vi "SolutionCalculator (SubVI).vi"(3 "Iterative?":bool, 4 "Max Iteration Count":dbl=2.0, 5 "Base Run (matrix)":T1, 6 "Response Coefficients":cdb[][](array[numeric])) -> (0 "Max Residual":dbl, 1 "Correction Phase (radians)":T2, 2 "Correction Mag":T2)   [LabVIEW 2010]
uses:
  <vilib>/Analysis/Matrix/Datatypes/ComplexMatrix.ctl
  <vilib>/Analysis/Matrix/Datatypes/RealMatrix.ctl
  <vilib>/Analysis/baseanly.llb/Complex A x B.vi
  <vilib>/Analysis/baseanly.llb/Complex Inverse Matrix.vi
  <vilib>/Analysis/Matrix/Numeric/Add/Add - CM,CM.vi
  <vilib>/Analysis/Matrix/Numeric/Conversions/Matrix To Array - CM.vi
  <vilib>/Analysis/Matrix/Numeric/Complex/Complex To Polar - CM.vi
  <vilib>/Analysis/Matrix/Numeric/Absolute Value/Absolute Value - CM.vi
  <vilib>/Analysis/NI_AALBase.lvlib
  <vilib>/Analysis/Matrix/NI_Matrix.lvlib
panel:
  out "A x B":T1
  out "Epsilon/R":T2
  out "Epsilon":T1
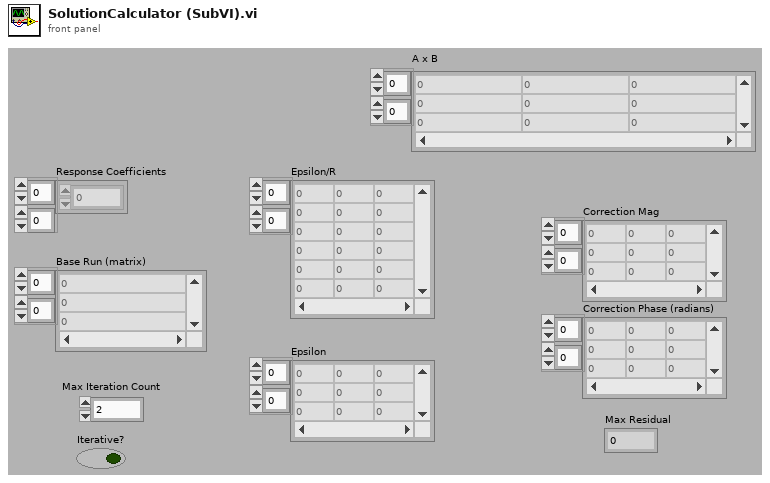
[diagram p1: front panel]
types:
  T1 = typedef "NI_Matrix.lvlib/ComplexMatrix.ctl" = cdb[][]
  T2 = typedef "NI_Matrix.lvlib/RealMatrix.ctl" = dbl[][]
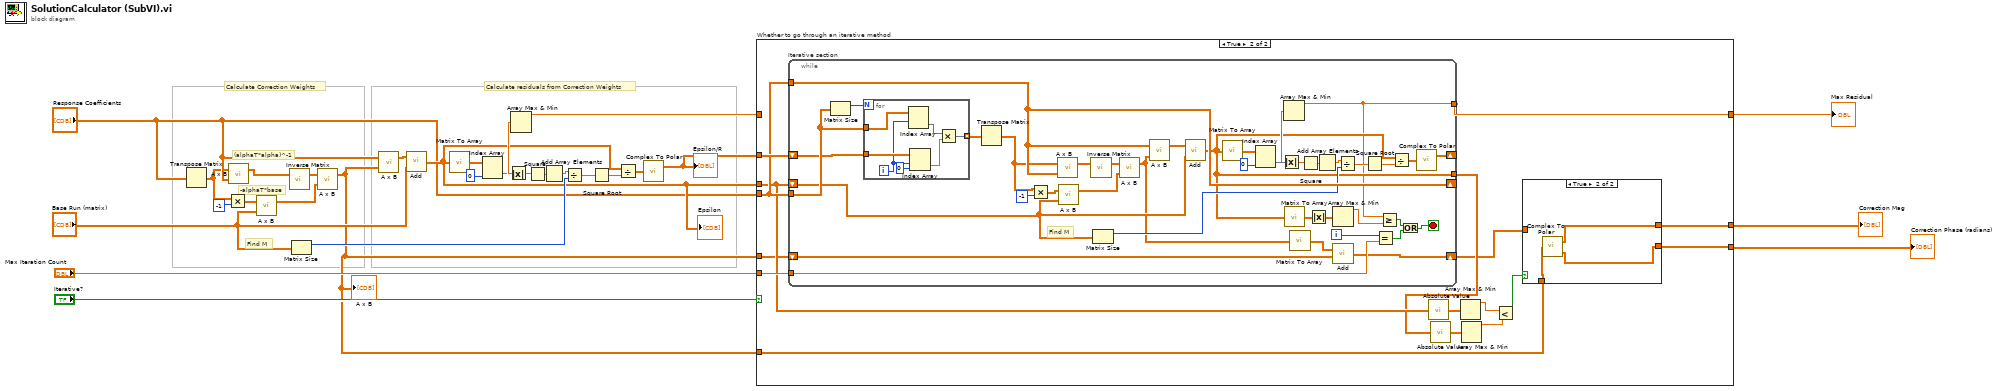
[diagram p0: block diagram]
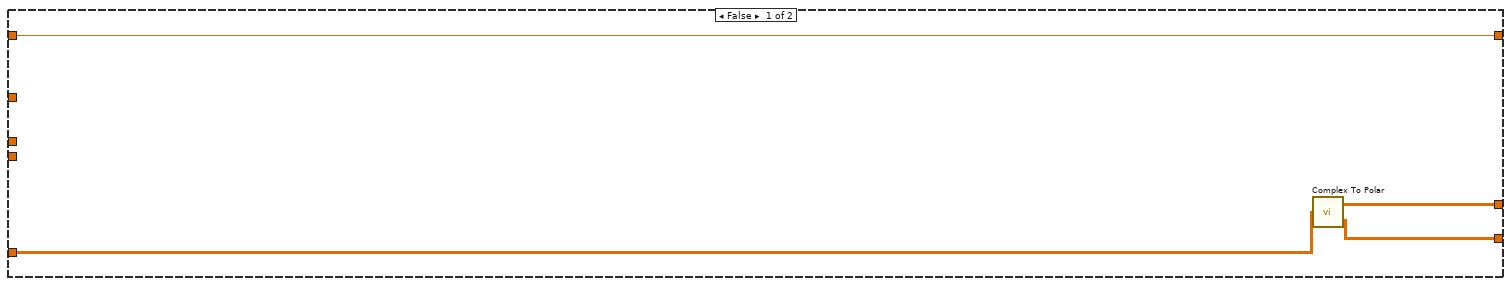
[diagram p2: hidden frame]
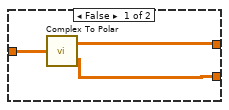
[diagram p3: hidden frame]
diagram:
  # "Calculate residuals from Correction Weights"
  # "Calculate Correction Weights"
  # "-alphaT*base"
  # "(alphaT*alpha)^-1"
  # "Find M"
  n1 = Transpose Matrix(1:"Response Coefficients") -> (0:w4:cdb[][])
  n2 = Multiply ("Multiply.vi")(x=w4, y=-1) -> (x*y=w3:cdb[][])
  n3 = call-poly <vilib>:"A x B.vi"("B"="Response Coefficients", "A"=w4) -> ("A x B"=w2:T1)  [unwired: 1 out]
  n4 = call-poly <vilib>:"A x B.vi"("B"="Base Run (matrix)", "A"=w3) -> ("A x B"=w16:T1)  [unwired: 1 out]
  n5 = call-poly <vilib>:"Inverse Matrix.vi"("Input Matrix"=w2) -> ("Inverse Matrix"=w15:T1)  [unwired: 1 in, 1 out]
  n6 = Matrix Size(0:"Base Run (matrix)") -> (1:w28:i32)  [unwired: 1 out]
  n7 = call-poly <vilib>:"A x B.vi"("B"=w16, "A"=w15) -> ("A x B"=w1:T1)  [unwired: 1 out]
  "A x B" <- w1
  n8 = call-poly <vilib>:"A x B.vi"("B"=w1, "A"="Response Coefficients") -> ("A x B"=w17:T1)  [unwired: 1 out]
  n9 = call-poly <vilib>:"Add.vi"("Complex Matrix B"="Base Run (matrix)", "Complex Matrix A"=w17) -> ("A + B"=w12:T1)
  "Epsilon" <- w12
  n10 = call-poly <vilib>:"Matrix To Array.vi"("Complex Matrix"=w12) -> ("Complex 2D Array"=w18:cdb[][])
  n11 = Index Array(array=w18, index (col)=0 ("disabled index (col)")) -> (element=w25:cdb[])  [unwired: 1 in]
  n12 = Absolute Value(x=w25) -> (abs(x)=w26:dbl[])
  n13 = Array Max & Min(array=w26) -> (max value=w9:dbl)  [unwired: 3 out]
  n14 = Square(x=w26) -> (x^2=w20:dbl[])
  n15 = Add Array Elements(numeric array=w20) -> (sum=w21:dbl)
  n16 = Divide(x=w21, y=w28) -> (x/y=w22:dbl)
  n17 = Square Root(x=w22) -> (sqrt(x)=w23:dbl)
  n18 = Divide(x=w12, y=w23) -> (x/y=w24:T1)
  n19 = call-poly <vilib>:"Complex To Polar.vi"("Complex Matrix r*e^iQ"=w24) -> ("Modulus r"=w13:T2)  [unwired: 1 out]
  "Epsilon/R" <- w13
  n20 = case "Whether to go through an iterative method" shown="True" "Iterative?" {
    tunnel: "Max Iteration Count" -> [_ w48]
    tunnel: w13 -> [_ w47]
    tunnel: w12 -> [_ w39]
    tunnel: "Response Coefficients" -> [_ w46]
    tunnel: w9 -> [w32 _]
    tunnel: [w32 w45] -> w8
    tunnel: w1 -> [w31 w34]
    tunnel: [w30 w36] -> w7
    tunnel: [w29 w35] -> w6
    tunnel: w1 -> [_ w33]
    frame False {
      n21 = call-poly <vilib>:"Complex To Polar.vi"("Complex Matrix r*e^iQ"=w31) -> ("Modulus r"=w30:T2, "Argument Q"=w29:T2)
    }
    frame True {
      n22 = while "Iterative section" {
        tunnel: w46 -> [w90]
        shift-right: [w63] -> _
        shift-left: w47 -> [w89]
        shift-right: [w64] -> _
        shift-left: w39 -> [w65]
        shift-right: [w79] -> w37
        shift-left: w34 -> [w78]
        tunnel: w48 -> [w80]
        tunnel: w46 -> [w64]
        tunnel: [w59] -> w45
        tunnel: [w61] -> w38
        i -> [w82]
        stop <- w81 stop-if-true
        # "Find M"
        n23 = Matrix Size(0:w90) -> (1:w92:i32)  [unwired: 1 out]
        n24 = for {
          N: w92 -> [_]
          tunnel: w90 -> [w96]
          tunnel: w89 -> [w99]
          tunnel: [w97] -> w91 mode=indexing
          i -> [w93]
          n25 = Index Array(array=w96, index (row)=w93) -> (element=w95:cdb[])  [unwired: 1 in]
          n26 = Index Array(array=w99, index (row)=w93, index (col)=0 ("disabled index (col)")) -> (element=w98:dbl)
          n27 = Multiply(x=w95, y=w98) -> (x*y=w97:cdb[])
        }
        n28 = Transpose Matrix(1:w91) -> (0:w55:cdb[][])
        n29 = Multiply ("Multiply.vi")(x=w55, y=-1) -> (x*y=w57:cdb[][])
        n30 = call-poly <vilib>:"A x B.vi"("B"=w64, "A"=w55) -> ("A x B"=w56:T1)  [unwired: 1 out]
        n31 = call-poly <vilib>:"A x B.vi"("B"=w65, "A"=w57) -> ("A x B"=w76:T1)  [unwired: 1 out]
        n32 = call-poly <vilib>:"Inverse Matrix.vi"("Input Matrix"=w56) -> ("Inverse Matrix"=w77:T1)  [unwired: 1 in, 1 out]
        n33 = Matrix Size(0:w65) -> (1:w62:i32)  [unwired: 1 out]
        n34 = call-poly <vilib>:"A x B.vi"("B"=w76, "A"=w77) -> ("A x B"=w60:T1)  [unwired: 1 out]
        n35 = call-poly <vilib>:"A x B.vi"("B"=w60, "A"=w64) -> ("A x B"=w75:T1)  [unwired: 1 out]
        n36 = call-poly <vilib>:"Add.vi"("Complex Matrix B"=w65, "Complex Matrix A"=w75) -> ("A + B"=w61:T1)
        n37 = call-poly <vilib>:"Matrix To Array.vi"("Complex Matrix"=w61) -> ("Complex 2D Array"=w74:cdb[][])
        n38 = Index Array(array=w74, index (col)=0 ("disabled index (col)")) -> (element=w67:cdb[])  [unwired: 1 in]
        n39 = Absolute Value(x=w67) -> (abs(x)=w66:dbl[])
        n40 = Array Max & Min(array=w66) -> (max value=w59:dbl)  [unwired: 3 out]
        n41 = call-poly <vilib>:"Matrix To Array.vi"("Complex Matrix"=w61) -> ("Complex 2D Array"=w84:cdb[][])
        n42 = call-poly <vilib>:"Matrix To Array.vi"("Complex Matrix"=w60) -> ("Complex 2D Array"=w83:cdb[][])
        n43 = Square(x=w66) -> (x^2=w72:dbl[])
        n44 = Absolute Value(x=w84) -> (abs(x)=w85:dbl[][])
        n45 = Add Array Elements(numeric array=w72) -> (sum=w71:dbl)
        n46 = Array Max & Min(array=w85) -> (max value=w88:dbl)  [unwired: 3 out]
        n47 = call-poly <vilib>:"Add.vi"("Complex Matrix B"=w78, "Complex Matrix A"=w83) -> ("A + B"=w79:T1)
        n48 = Divide(x=w71, y=w62) -> (x/y=w70:dbl)
        n49 = Square Root(x=w70) -> (sqrt(x)=w69:dbl)
        n50 = Equal?(x=w82, y=w80) -> (x = y?=w87:bool)
        n51 = Greater Or Equal?(x=w59, y=w88) -> (x >= y?=w86:bool)
        n52 = Divide(x=w61, y=w69) -> (x/y=w68:T1)
        n53 = Or(x=w86, y=w87) -> (x .or. y?=w81:bool)
        n54 = call-poly <vilib>:"Complex To Polar.vi"("Complex Matrix r*e^iQ"=w68) -> ("Modulus r"=w63:T2)  [unwired: 1 out]
      }
      n55 = call-poly <vilib>:"Absolute Value.vi"("Complex Matrix A"=w39) -> ("|A|"=w41:T2)
      n56 = call-poly <vilib>:"Absolute Value.vi"("Complex Matrix A"=w38) -> ("|A|"=w42:T2)
      n57 = Array Max & Min(array=w41) -> (max value=w43:dbl)  [unwired: 3 out]
      n58 = Array Max & Min(array=w42) -> (max value=w44:dbl)  [unwired: 3 out]
      n59 = Less?(x=w43, y=w44) -> (x < y?=w40:bool)
      n60 = case shown="True" w40 {
        tunnel: w37 -> [w50 _]
        tunnel: [w51 w54] -> w36
        tunnel: [w49 w52] -> w35
        tunnel: w33 -> [_ w53]
        frame False {
          n61 = call-poly <vilib>:"Complex To Polar.vi"("Complex Matrix r*e^iQ"=w50) -> ("Modulus r"=w51:T2, "Argument Q"=w49:T2)
        }
        frame True {
          n62 = call-poly <vilib>:"Complex To Polar.vi"("Complex Matrix r*e^iQ"=w53) -> ("Modulus r"=w54:T2, "Argument Q"=w52:T2)
        }
      }
    }
  }
  "Max Residual" <- w8
  "Correction Mag" <- w7
  "Correction Phase (radians)" <- w6
